vi "GetImageRes.vi"(8 "error in (no error)":errorcluster, 11 "Image":T1) -> (0 "valid Image":bool, 1 "Image Area:Size:All Elements":cluster{"Width":u32, "Height":u32}, 2 "Y Resolution":i32, 3 "X Resolution":i32, 4 "error out":errorcluster)   [LabVIEW 2013]
uses:
  <vilib>/vision/Image Controls.llb/IMAQ Image.ctl
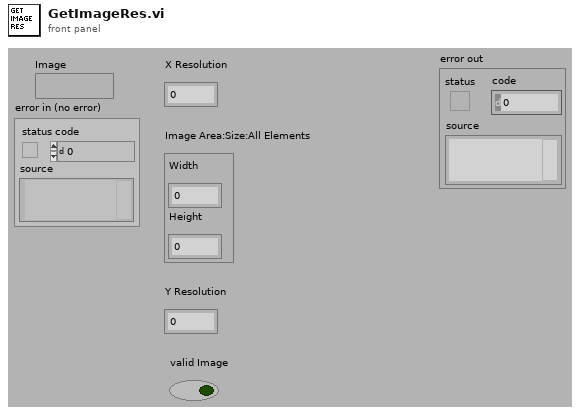
[diagram p1: front panel]
types:
  T1 = typedef "IMAQ Image.ctl" = refnum<image>
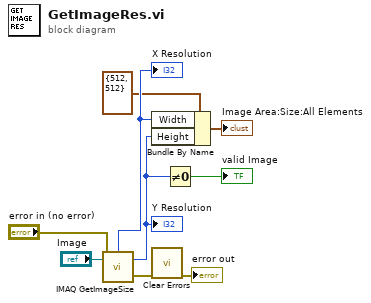
[diagram p0: block diagram]
diagram:
  n1 = call "IMAQ GetImageSize"("Image"="Image", "error in (no error)"="error in (no error)") -> ("Y Resolution"=w8:i32, "X Resolution"=w7:i32, "error out"=w6:errorcluster)  [unwired: 2 in]
  "Y Resolution" <- w8
  "X Resolution" <- w7
  n2 = Bundle By Name(cluster=cluster{"Width":u32, "Height":u32} {"Width"=512, "Height"=512} ("Image Area:Size:All Elements"), "Width"=w7, "Height"=w8) -> (→"Image Area:Size:All Elements":cluster{"Width":u32, "Height":u32})
  n3 = call <vilib>:"Clear Errors.vi"("error in (no error)"=w6) -> ("error out"=→"error out":errorcluster)  [unwired: 6 in]
  n4 = Not Equal To 0?(x=w8) -> (x != 0?=→"valid Image":bool)
